vi "Terminate.vi"(8 "error in (no error)":errorcluster, 11 "WAMP Client in":refnum<class "WAMP Client.lvclass">) -> (0 "error out":errorcluster, 3 "WAMP Client out":refnum<class "WAMP Client.lvclass">)   [LabVIEW 2020, in "wamplv.lvlib" / "WAMP Client.lvclass"]
uses:
  <userlib>/wamplv/WAMP Client/WAMP Client.lvclass
  <userlib>/wamplv/WAMP Client/TypeDef/Internal Daemon Termination Loop Msg.ctl
  <userlib>/wamplv/WAMP Client/WAMP Client.lvclass/WAMP Client.ctl
  <vilib>/JDP Science/JSONtext/Get Array Elements.vi
  <userlib>/wamplv/Comm Handlers/ICommHandler/ICommHandler.lvclass
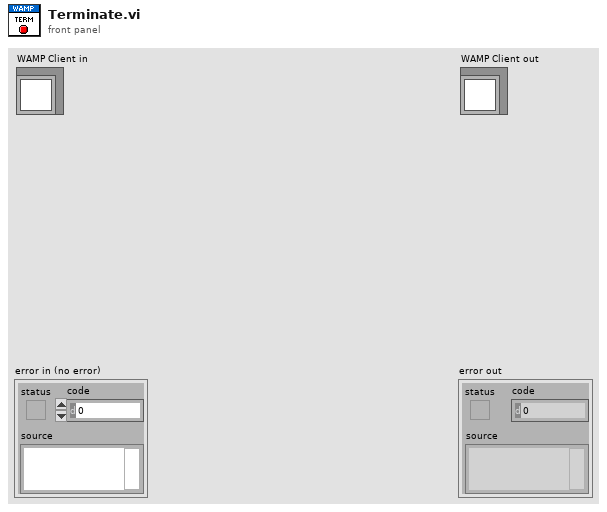
[diagram p1: front panel]
types:
  T1 = typedef "wamplv.lvlib/WAMP Client.lvclass/Termination Reason.ctl" = cluster{"Reason":T2, "Reason URI":string, "Message":string}
  T2 = typedef "wamplv.lvlib/WAMP Client.lvclass/Termination Reason Enum.ctl" = enum16{"Goodbye Received", "Abort Received", "Send Goodbye", "Send Abort", "Read Loop Failure", "Write Loop Failure", "Message Loop Failure"}
  T3 = typedef "wamplv.lvlib/WAMP Client.lvclass/Internal Daemon Termination Loop Msg.ctl" = enum16{"Send Goodbye and Wait For Response", "Send Goodbye and Terminate", "Wait for Goodbye", "Send Abort", "Terminate"}
  T4 = typedef "wamplv.lvlib/WAMP Client.lvclass/WAMP Message Codes.ctl" = u16
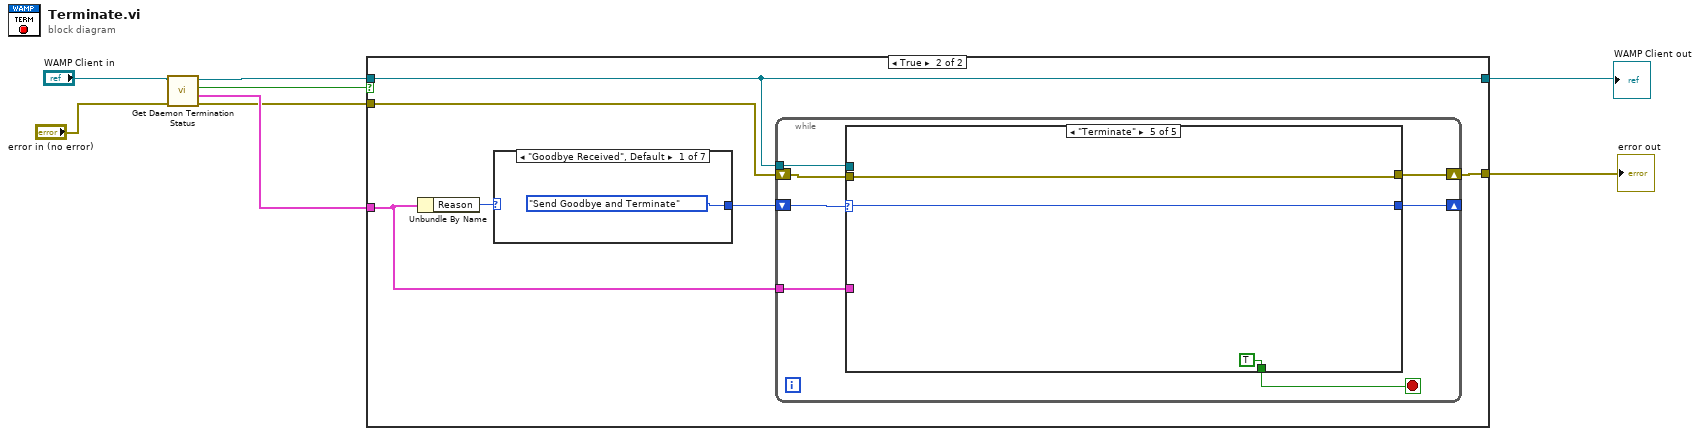
[diagram p0: block diagram]
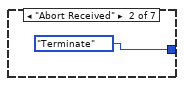
[diagram p3: hidden frame]
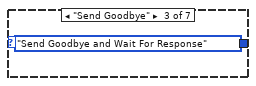
[diagram p4: hidden frame]
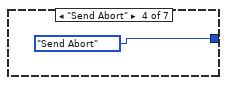
[diagram p5: hidden frame]
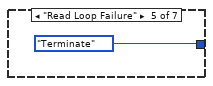
[diagram p6: hidden frame]
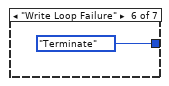
[diagram p7: hidden frame]
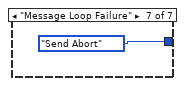
[diagram p8: hidden frame]
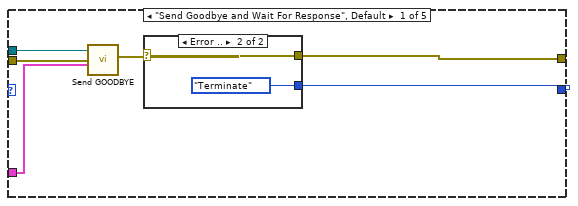
[diagram p9: hidden frame]
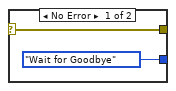
[diagram p10: hidden frame]
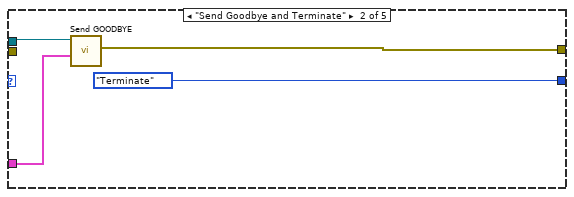
[diagram p11: hidden frame]
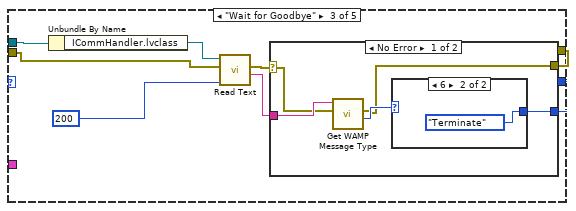
[diagram p12: hidden frame]
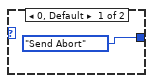
[diagram p13: hidden frame]
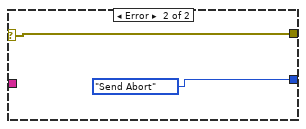
[diagram p14: hidden frame]
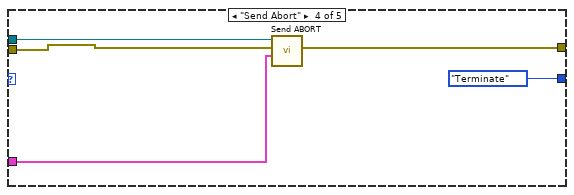
[diagram p15: hidden frame]
diagram:
  n1 = call <userlib>:"Get Daemon Termination Status.vi"("error in (no error)"="error in (no error)", "WAMP Client in"="WAMP Client in") -> ("error out"=w2:errorcluster, "Termination Reason"=w5:T1, "Terminate?"=w3:bool, "WAMP Client out"=w7:refnum<class "WAMP Client.lvclass">)  [unwired: 6 in]
  n2 = case shown="True" w3 {
    tunnel: w7 -> [w9 w11]
    tunnel: w5 -> [_ w14]
    tunnel: [w10 w13] -> w4
    tunnel: w2 -> [w10 w12]
    tunnel: [w9 w11] -> w1
    frame False {
    }
    frame True {
      n3 = Unbundle By Name(w14) -> ("Reason"=w15:T2)
      n4 = case shown="\"Goodbye Received\", Default" w15 {
        tunnel: [Internal_Daemon_Termination_Loop_Msg."Send Goodbye and Terminate" ("Termination Loop Msg") Internal_Daemon_Termination_Loop_Msg."Terminate" ("Termination Loop Msg") Internal_Daemon_Termination_Loop_Msg."Send Goodbye and Wait For Response" ("Termination Loop Msg") Internal_Daemon_Termination_Loop_Msg."Send Abort" ("Termination Loop Msg") Internal_Daemon_Termination_Loop_Msg."Terminate" ("Termination Loop Msg") Internal_Daemon_Termination_Loop_Msg."Terminate" ("Termination Loop Msg") Internal_Daemon_Termination_Loop_Msg."Send Abort" ("Termination Loop Msg")] -> w16
        frame "Goodbye Received", Default {
        }
        frame "Abort Received" {
        }
        frame "Send Goodbye" {
        }
        frame "Send Abort" {
        }
        frame "Read Loop Failure" {
        }
        frame "Write Loop Failure" {
        }
        frame "Message Loop Failure" {
        }
      }
      n5 = while {
        shift-right: [w27] -> _
        shift-left: w16 -> [w30]
        tunnel: w11 -> [w29]
        tunnel: w14 -> [w28]
        shift-right: [w25] -> w13
        shift-left: w12 -> [w24]
        stop <- w26 stop-if-true
        n6 = case shown="\"Terminate\"" w30 {
          selector: w30 -> [_ _ _ _ w68]
          tunnel: w29 -> [w33 w44 w52 w66 _]
          tunnel: w28 -> [w31 w41 _ w62 _]
          tunnel: [w35 Internal_Daemon_Termination_Loop_Msg."Terminate" ("Termination Loop Msg") w47 Internal_Daemon_Termination_Loop_Msg."Terminate" ("Termination Loop Msg") w68] -> w27
          tunnel: [_ _ _ _ TRUE] -> w26
          tunnel: [w34 w42 w46 w64 w67] -> w25
          tunnel: w24 -> [w32 _ w45 w63 w67]
          frame "Send Goodbye and Wait For Response", Default {
            n7 = call-dynamic "Send GOODBYE.vi"("Termination Reason"=w31, "error in (no error)"=w32, "WAMP Client in"=w33) -> ("error out"=w36:errorcluster)  [unwired: 7 in, 1 out]
            n8 = case shown="Error .." w36 {
              selector: w36 -> [w37 w39]
              tunnel: [Internal_Daemon_Termination_Loop_Msg."Wait for Goodbye" ("Termination Loop Msg") Internal_Daemon_Termination_Loop_Msg."Terminate" ("Termination Loop Msg")] -> w35
              tunnel: [w37 w39] -> w34
              frame No Error {
              }
              frame Error {
              }
            }
          }
          frame "Send Goodbye and Terminate" {
            n9 = call-dynamic "Send GOODBYE.vi"("Termination Reason"=w41, "WAMP Client in"=w44) -> ("error out"=w42:errorcluster)  [unwired: 8 in, 1 out]
          }
          frame "Wait for Goodbye" {
            n10 = Unbundle By Name(w52) -> ("ICommHandler.lvclass"=w51:refnum<class "ICommHandler.lvclass">)
            n11 = call-dynamic "Read Text.vi"("timeout ms (5000)"=200, "error in (no error)"=w45, "ICommHandler in"=w51) -> ("String"=w48:string, "error out"=w49:errorcluster)  [unwired: 4 in, 1 out]
            n12 = case shown="No Error" w49 {
              selector: w49 -> [w54 w60]
              tunnel: w48 -> [w57 _]
              tunnel: [w55 Internal_Daemon_Termination_Loop_Msg."Send Abort" ("Termination Loop Msg")] -> w47
              tunnel: [w53 w60] -> w46
              frame No Error {
                n13 = call <userlib>:"Get WAMP Message Type.vi"("error in (no error)"=w54, "JSON"=w57) -> ("Message Codes"=w56:T4, "error out"=w53:errorcluster)  [unwired: 6 in, 2 out]
                n14 = case shown="6" w56 {
                  tunnel: [Internal_Daemon_Termination_Loop_Msg."Send Abort" ("Termination Loop Msg") Internal_Daemon_Termination_Loop_Msg."Terminate" ("Termination Loop Msg")] -> w55
                  frame 0, Default {
                  }
                  frame 6 {
                  }
                }
              }
              frame Error {
              }
            }
          }
          frame "Send Abort" {
            n15 = call-dynamic "Send ABORT.vi"("Abort Request"=w62, "error in (no error)"=w63, "WAMP Client in"=w66) -> ("error out"=w64:errorcluster)  [unwired: 7 in, 1 out]
          }
          frame "Terminate" {
          }
        }
      }
    }
  }
  "error out" <- w4
  "WAMP Client out" <- w1
